vi "Validate Pairing.vi"(8 "error in (no error)":errorcluster, 10 "E2E node 2":refnum<data-value>, 11 "E2E node 1":refnum<data-value>) -> (0 "error out":errorcluster, 2 "E2E node 2 out":refnum<data-value>, 3 "E2E node 1 out":refnum<data-value>)   [LabVIEW 2015, in "E2E Tag Exchange editor node.lvclass"]
uses:
  E2E Tag Exchange editor node.lvclass
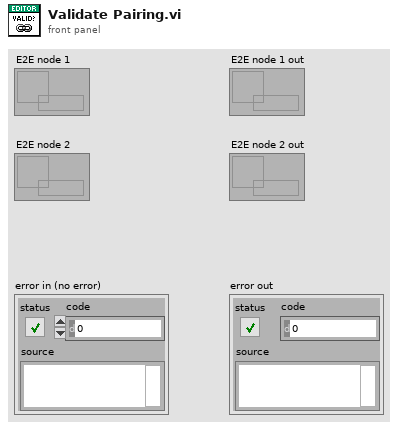
[diagram p1: front panel]
types:
  T1 = typedef "E2E Tag Exchange configuration.lvclass/Runtime Implementation.ctl" = enum16{"RT FIFO", "UDP"}
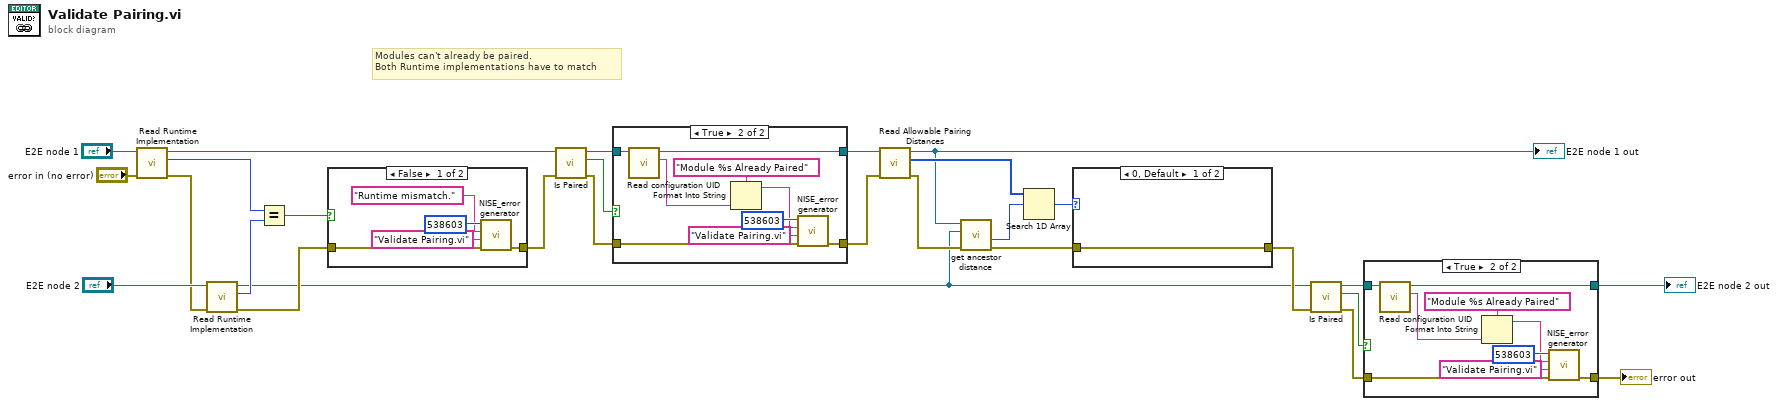
[diagram p0: block diagram]
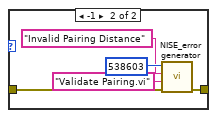
[diagram p2: hidden frame]
diagram:
  # "Modules can't already be paired.\nBoth Runtime implementations have to match"
  n1 = call "Read Runtime Implementation.vi"("error in (no error)"="error in (no error)", "E2E editor node in"="E2E node 1") -> ("error out"=w23:errorcluster, "Runtime Implementation"=w28:T1, "E2E editor node out"=w24:refnum<data-value>)  [unwired: 7 in]
  n2 = call "Read Runtime Implementation.vi"("error in (no error)"=w23, "E2E editor node in"="E2E node 2") -> ("error out"=w20:errorcluster, "Runtime Implementation"=w27:T1, "E2E editor node out"=w1:refnum<data-value>)  [unwired: 7 in]
  n3 = Equal?(x=w28, y=w27) -> (x = y?=w21:bool)
  n4 = case shown="False" w21 {
    tunnel: w20 -> [w32 w34]
    tunnel: [w31 w34] -> w19
    frame False {
      n5 = call <vilib>:"NISE_error generator.vi"("error in"=w32, "source"="Validate Pairing.vi", "append error message"="Runtime mismatch.", "error code (0)"=538603) -> ("error out"=w31:errorcluster)  [unwired: 5 in]
    }
    frame True {
    }
  }
  n6 = call "Is Paired.vi"("error in (no error)"=w19, "E2E editor node in"=w24) -> ("error out"=w18:errorcluster, "Paired?"=w17:bool, "E2E editor node out"=w16:refnum<data-value>)  [unwired: 7 in]
  n7 = case shown="True" w17 {
    tunnel: w18 -> [w36 w44]
    tunnel: [w36 w43] -> w7
    tunnel: w16 -> [w35 w41]
    tunnel: [w35 w37] -> w12
    frame False {
    }
    frame True {
      n8 = call "Read configuration UID.vi"("E2E editor node in"=w41) -> ("Module UID"=w39:string, "E2E editor node out"=w37:refnum<data-value>)  [unwired: 8 in, 1 out]
      n9 = Format Into String(format string="Module %s Already Paired" ("append error message"), w39) -> (resulting string=w38:string)  [unwired: 2 in, 1 out]
      n10 = call <vilib>:"NISE_error generator.vi"("error in"=w44, "source"="Validate Pairing.vi", "append error message"=w38, "error code (0)"=538603) -> ("error out"=w43:errorcluster)  [unwired: 5 in]
    }
  }
  n11 = call "Read Allowable Pairing Distances.vi"("error in (no error)"=w7, "E2E editor node in"=w12) -> ("error out"=w6:errorcluster, "Allowable Pairing Distances"=w11:i32[], "E2E editor node out"=w8:refnum<data-value>)  [unwired: 7 in]
  "E2E node 1 out" <- w8
  n12 = call "get ancestor distance.vi"("error in (no error)"=w6, "node 2"=w1, "node 1"=w8) -> ("error out"=w5:errorcluster, "Degree out"=w10:i32)  [unwired: 5 in, 2 out]
  n13 = Search 1D Array(1D array=w11, element=w10) -> (index of element=w4:i32)  [unwired: 1 in]
  n14 = case shown="0, Default" w4 {
    tunnel: w5 -> [w46 w50]
    tunnel: [w46 w49] -> w3
    frame 0, Default {
    }
    frame -1 {
      n15 = call <vilib>:"NISE_error generator.vi"("error in"=w50, "source"="Validate Pairing.vi", "append error message"="Invalid Pairing Distance", "error code (0)"=538603) -> ("error out"=w49:errorcluster)  [unwired: 5 in]
    }
  }
  n16 = call "Is Paired.vi"("error in (no error)"=w3, "E2E editor node in"=w1) -> ("error out"=w14:errorcluster, "Paired?"=w13:bool, "E2E editor node out"=w15:refnum<data-value>)  [unwired: 7 in]
  n17 = case shown="True" w13 {
    tunnel: w14 -> [w53 w61]
    tunnel: [w53 w60] -> w2
    tunnel: w15 -> [w52 w58]
    tunnel: [w52 w54] -> w9
    frame False {
    }
    frame True {
      n18 = call "Read configuration UID.vi"("E2E editor node in"=w58) -> ("Module UID"=w56:string, "E2E editor node out"=w54:refnum<data-value>)  [unwired: 8 in, 1 out]
      n19 = Format Into String(format string="Module %s Already Paired" ("append error message"), w56) -> (resulting string=w55:string)  [unwired: 2 in, 1 out]
      n20 = call <vilib>:"NISE_error generator.vi"("error in"=w61, "source"="Validate Pairing.vi", "append error message"=w55, "error code (0)"=538603) -> ("error out"=w60:errorcluster)  [unwired: 5 in]
    }
  }
  "E2E node 2 out" <- w9
  "error out" <- w2
